vi "用户信息加密解密.vi"(5 "原始字符串_in":string, 6 "加密字符串_in":string, 7 "T解密-F加密":bool=TRUE) -> (1 "加密字符串_out":string, 2 "原始字符串_out":string)   [LabVIEW 2018]
panel:
  out "无符号字节数组 3":u8[](array[numeric]) format="%08b"
  out "无符号字节数组 2":u8[](array[numeric]) format="%08b"
  out "x循环左移y位":u8[](array[numeric])
  out "无符号字节数组":u8[](array[numeric])
  # "怎么显示的？"
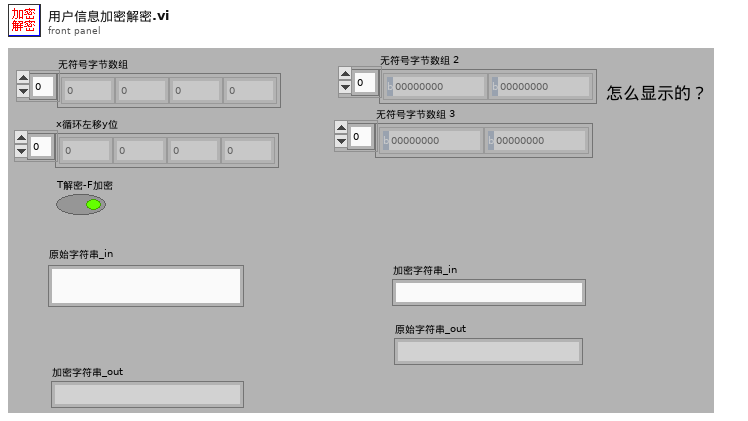
[diagram p1: front panel]
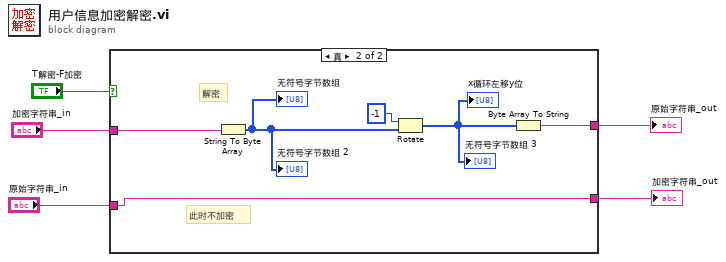
[diagram p0: block diagram]
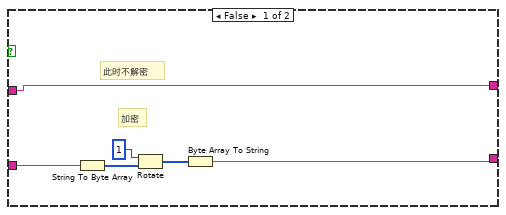
[diagram p2: hidden frame]
diagram:
  n1 = case shown="真" "T解密-F加密" {
    tunnel: [w11 w16] -> w5
    tunnel: "加密字符串_in" -> [w11 w14]
    tunnel: "原始字符串_in" -> [w7 w15]
    tunnel: [w6 w15] -> w1
    frame False {
      # "加密"
      # "此时不解密"
      n2 = String To Byte Array(string=w7) -> (unsigned byte array=w9:u8[])
      n3 = Rotate(1:w9, 2:i8 1 ("y")) -> (0:w8:u8[])
      n4 = Byte Array To String(unsigned byte array=w8) -> (string=w6:string)
    }
    frame True {
      # "此时不加密"
      # "解密"
      n5 = String To Byte Array(string=w14) -> (unsigned byte array=w12:u8[])
      "无符号字节数组" <- w12
      "无符号字节数组 2" <- w12
      n6 = Rotate(1:w12, 2:i8 -1 ("y")) -> (0:w13:u8[])
      "x循环左移y位" <- w13
      "无符号字节数组 3" <- w13
      n7 = Byte Array To String(unsigned byte array=w13) -> (string=w16:string)
    }
  }
  "原始字符串_out" <- w5
  "加密字符串_out" <- w1
